vi "Client Test.vi"() -> ()   [LabVIEW 2018]
uses:
  IOPub Messages/status Message/Status Content.ctl
  Shell Messages/kernel_info_request Message/kernel_info_request Message.lvclass
  IOPub Messages/status Message/status Message.lvclass
  Shell Messages/kernel_info_reply Message/kernel_info_reply Message.lvclass
  IOPub Messages/error Message/error Message.lvclass
  Shell Messages/execute_reply Message/execute_reply Message.lvclass
  C:/Users/gavin/Documents/LabVIEW Data/LabVIEW-Bits/Connectivity/Jupyter Client/Base Classes/Reply Message/Reply Message.lvclass
  IOPub Messages/stream Message/stream Message.lvclass
  IOPub Messages/execute_result Message/execute_result Message.lvclass
  C:/Users/gavin/Documents/LabVIEW Data/LabVIEW-Bits/Connectivity/Jupyter Client/IOPub Messages/display_data Message/display_data Message.lvclass
  Shell Messages/shutdown_request Message/shutdown_request Message.lvclass
  Shell Messages/execute_request Message/execute_request Message.lvclass
  48e361d1-6cf2-4824-8834-e089fd543d5e.vi
  48e361d1-6cf2-4824-8834-e089fd543d5e.vi/d7fca688-9f3d-45d2-96bd-b0b513891c02.vi
  48e361d1-6cf2-4824-8834-e089fd543d5e.vi/f5f7bd2d-65e3-4118-a998-9a6677903c6e.vi
  JuPyter_Client/public/Start Kernel and Connect.vi
  <userlib>/_OpenG.lib/lvdata/lvdata.llb/Set Data Name__ogtk.vi
  <userlib>/_OpenG.lib/lvdata/lvdata.llb/Array of VData to VCluster__ogtk.vi
  JuPyter_Client/JuPyter_Client.lvclass
  Base Classes/Message Class/Message Class.lvclass
panel:
  in  "Outputs":T1(tab)
  in  "Streams":enum32{"stdout", "stdeerr"}(tab)
  in  "Cl;ear stdout":bool
  out "Stdout":string
  in  "Cl;ear stderr":bool
  out "stderr":string
  in  "Clear Results":bool
  out "Results":string[](array[string])
  in  "Clear Message":bool
  out "Message Data":string
  in  "Variables to Watch":string[](array[string])
  in  "Enter":bool
  in  "Code":string
  in  "Exit":bool
  out "Language and Version":string
  out "status":T2
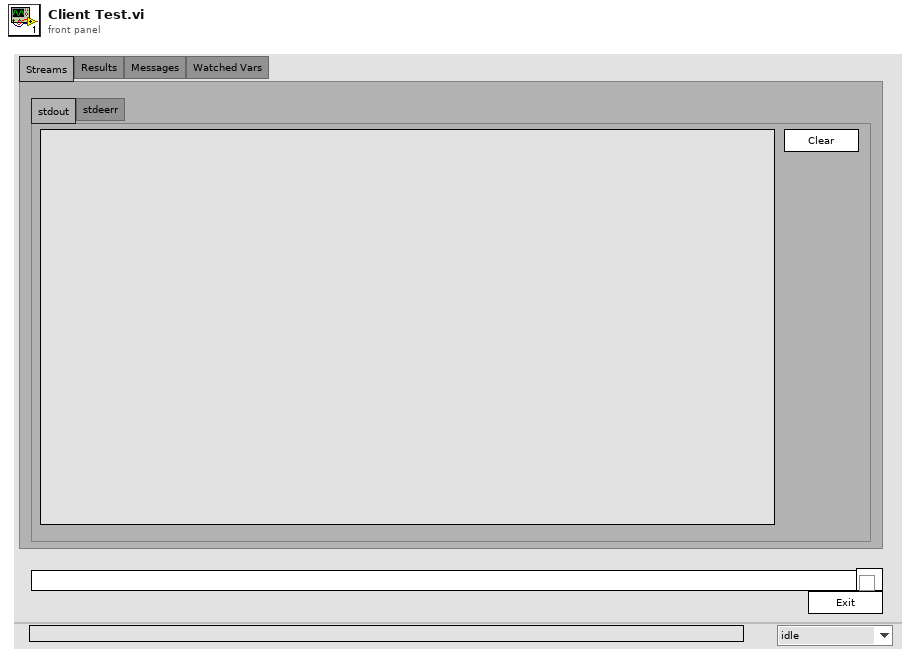
[diagram p1: front panel]
types:
  T1 = enum32{"Streams", "Results", "Messages", "Watched Vars"}
  T2 = typedef "ClientMessaging.lvlib/status Message.lvclass/Status Content.ctl" = enum16{"idle", "busy", "starting"}
  T3 = typedef "ClientMessaging.lvlib/Message Class.lvclass/header_dict.ctl" = cluster{"msg_id":string, "username":string, "session":string, "date":timestamp, "msg_type":string, "version":string}
  T4 = cluster{"ename":string, "evalue":string, "traceback":string[]}
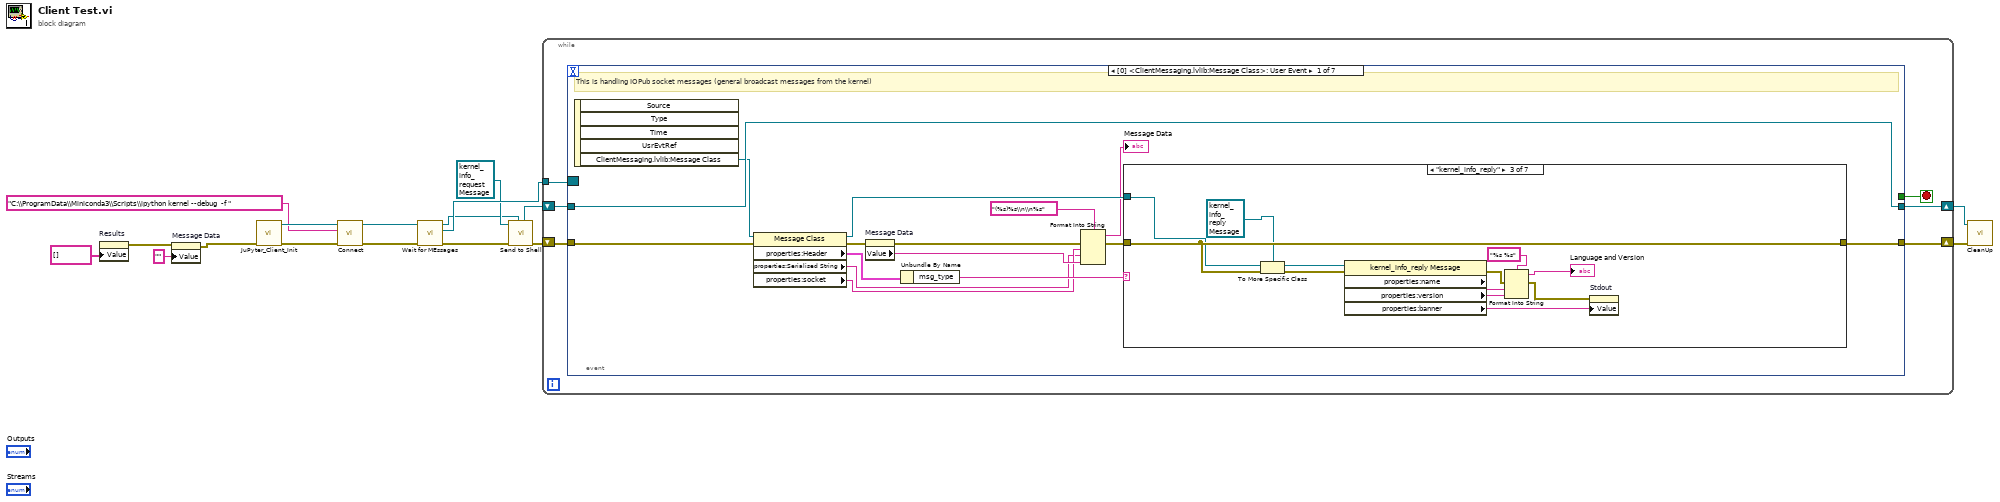
[diagram p0: block diagram]
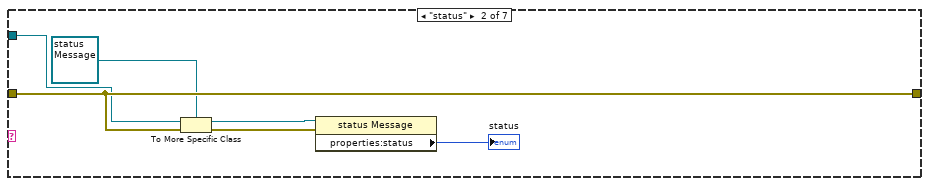
[diagram p3: hidden frame]
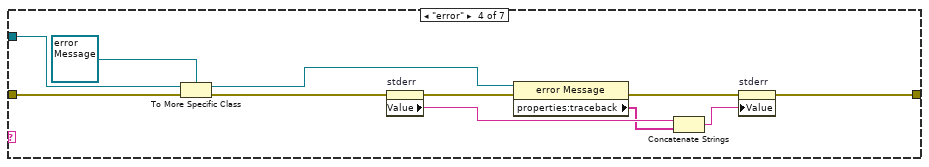
[diagram p4: hidden frame]
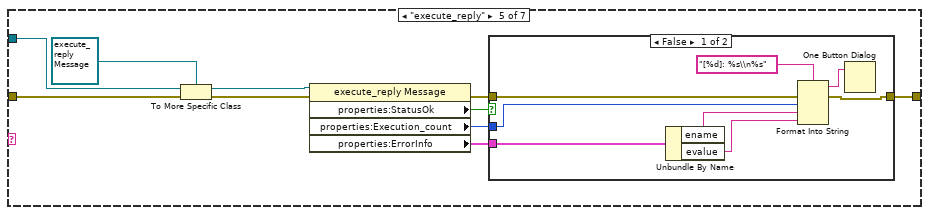
[diagram p5: hidden frame]
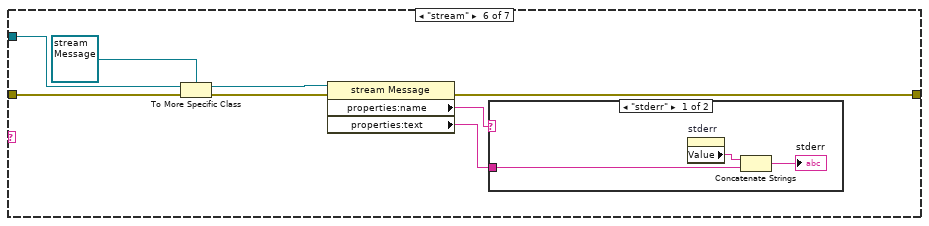
[diagram p7: hidden frame]
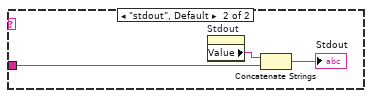
[diagram p8: hidden frame]
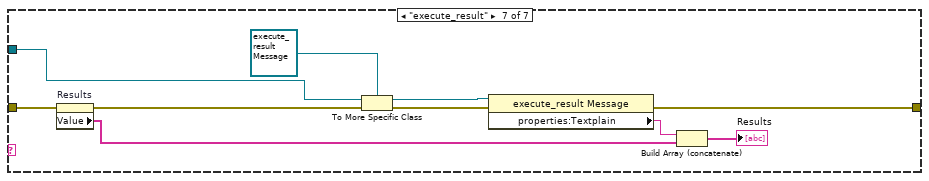
[diagram p9: hidden frame]
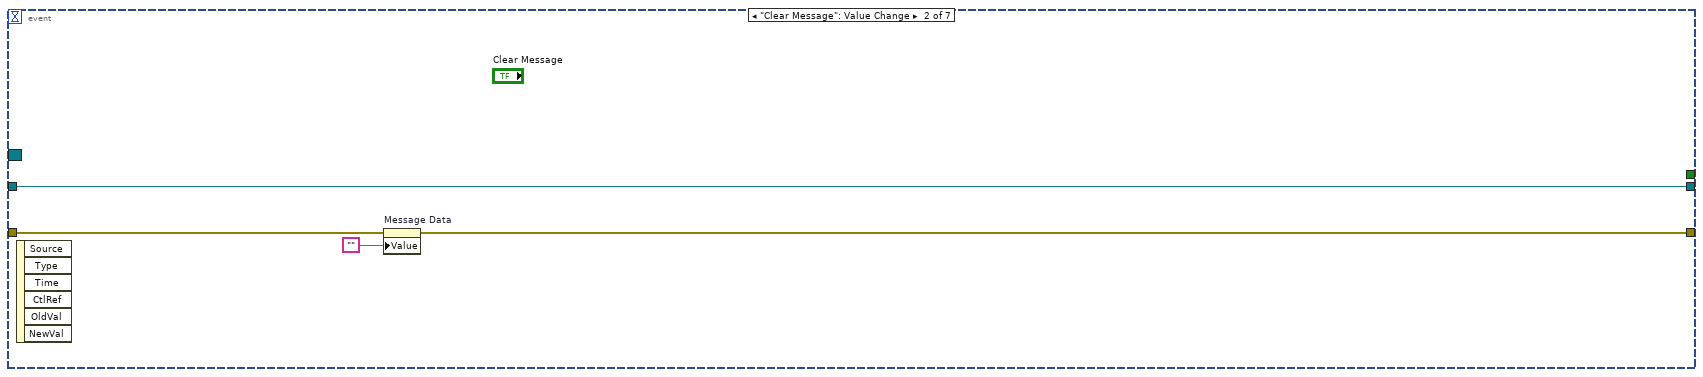
[diagram p10: hidden frame]
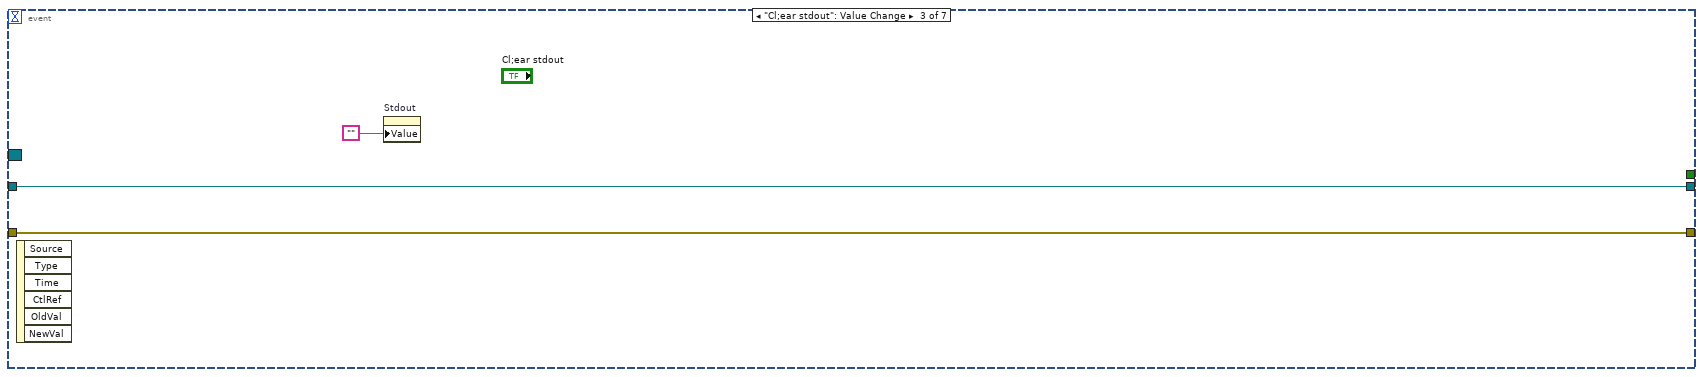
[diagram p11: hidden frame]
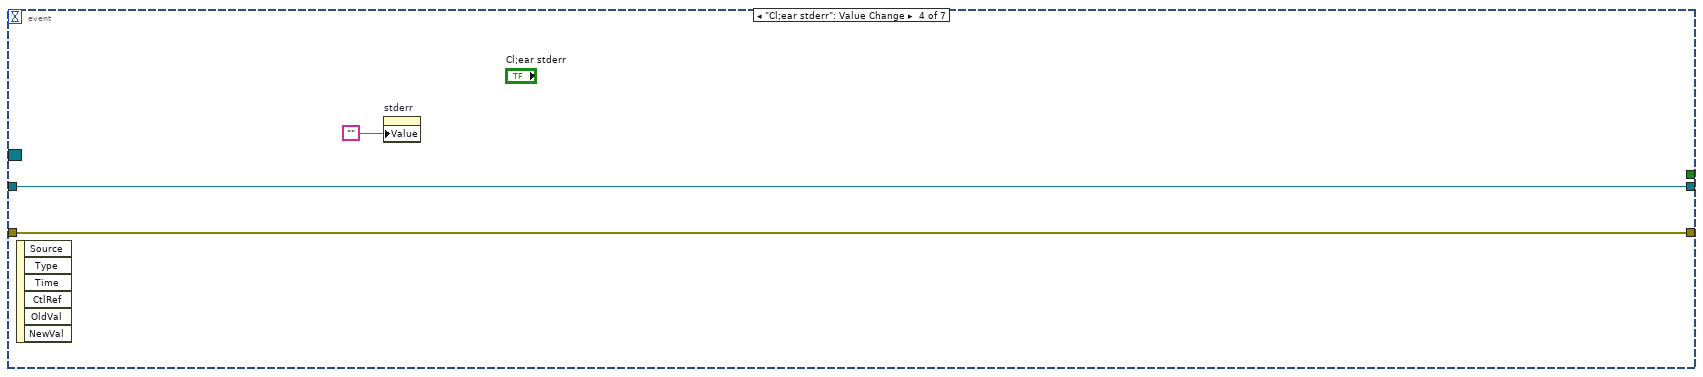
[diagram p12: hidden frame]
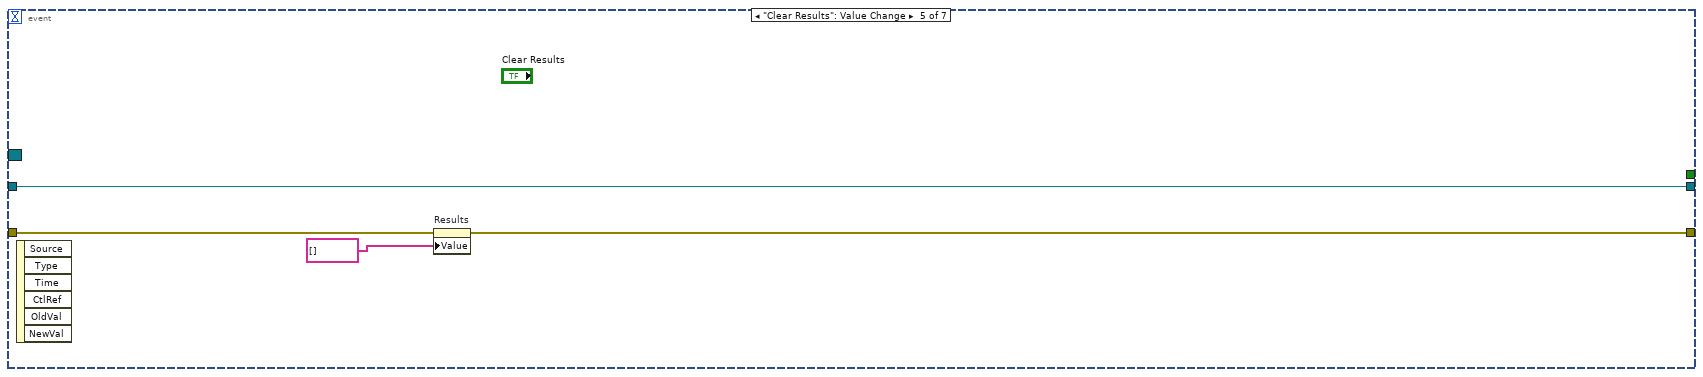
[diagram p13: hidden frame]
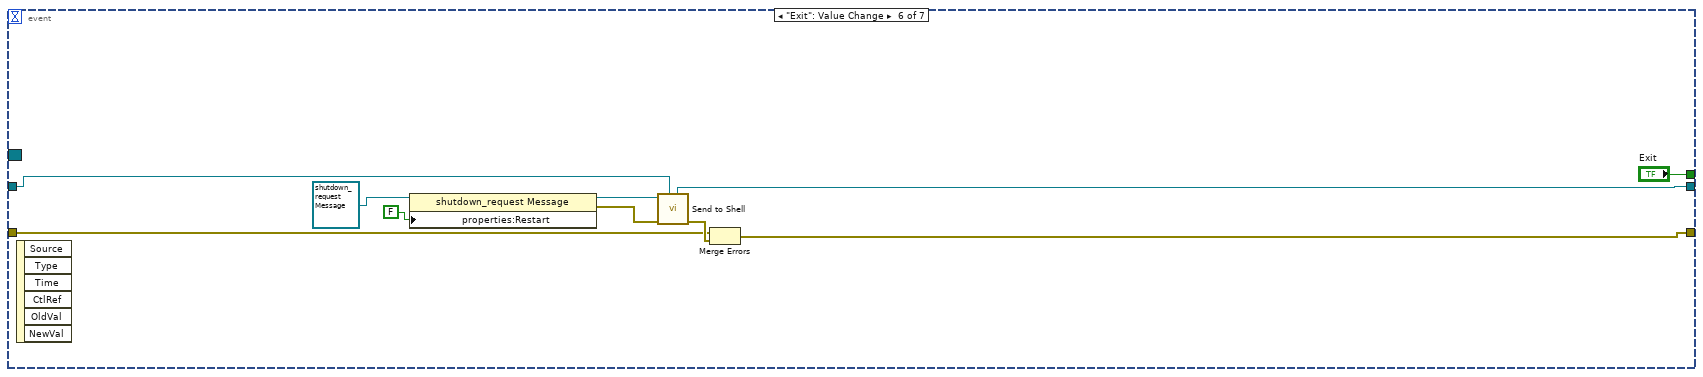
[diagram p14: hidden frame]
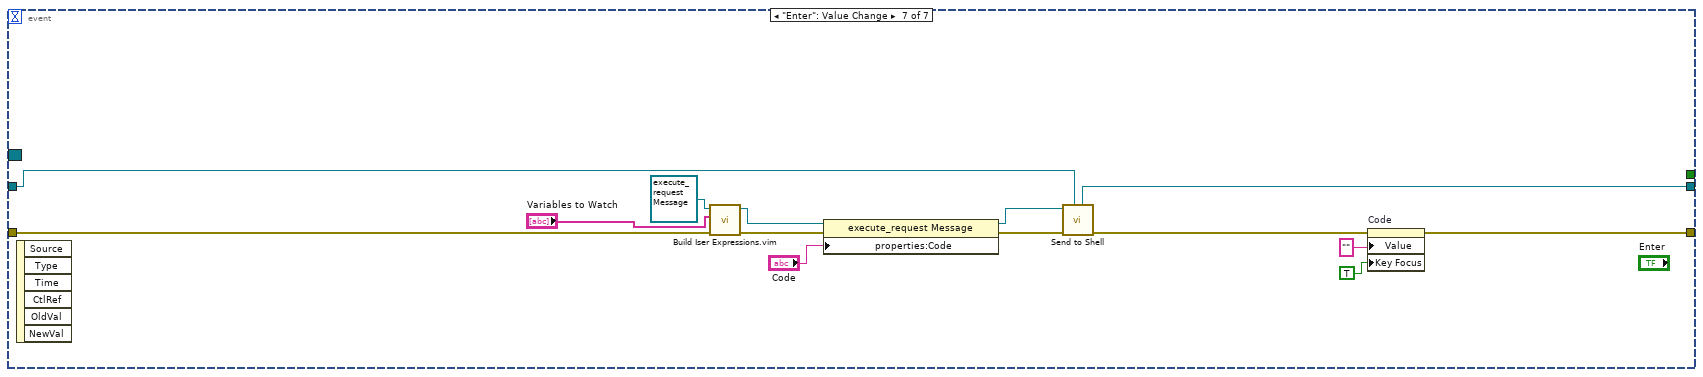
[diagram p15: hidden frame]
diagram:
  n1 = property on="Results" class="Arr (strict)"("Value"=string[] [] ("Results")) -> (error out=w2:errorcluster)  [unwired: 2 in, 1 out]
  n2 = property on="Message Data" class="Str"(error in=w2, "Value"="" ("Message Data")) -> (error out=w3:errorcluster)  [unwired: 1 in, 1 out]
  n3 = call "JuPyter_Client_Init.vi"("error in (no error)"=w3) -> ("error out"=w16:errorcluster, "object out"=w17:refnum<class "JuPyter_Client.lvclass">)  [unwired: 9 in]
  n4 = call-poly "Connect.vi"("error in (no error)"=w16, "Path to Kernel Command (IPython)"="C:\\ProgramData\\Miniconda3\\Scripts\\ipython kernel --debug  -f " ("Command"), "object in"=w17) -> ("error out"=w11:errorcluster, "object out"=w13:refnum<class "JuPyter_Client.lvclass">)  [unwired: 7 in]
  n5 = call-dynamic "Wait for MEssages.vi"("error in (no error)"=w11, "object in"=w13) -> ("error out"=w6:errorcluster, "Event Registration Refnum"=w10:refnum<event-registration>, "object out"=w8:refnum<class "JuPyter_Client.lvclass">)  [unwired: 7 in]
  n6 = call-dynamic "Send to Shell.vi"("Session In"=w8, "error in (no error)"=w6, "object in"=refnum<class "kernel_info_request Message.lvclass"> refnum ("ClientMessaging.lvlib:kernel_info_request Message")) -> ("error out"=w5:errorcluster, "Session Out"=w7:refnum<class "JuPyter_Client.lvclass">)  [unwired: 5 in, 2 out]
  n7 = while {
    shift-right: [w22] -> w15
    shift-left: w7 -> [w19]
    shift-right: [w20] -> w14
    shift-left: w5 -> [w23]
    tunnel: w10 -> [w18]
    stop <- w21 stop-if-true
    n8 = event shown="[0] <ClientMessaging.lvlib:Message Class>: User Event" {
      selector: w18 -> [_ _ _ _ _ _ _]
      dyn-events: _ -> [_ _ _ _ _ _ _]
      timeout: _ -> [_ _ _ _ _ _ _]
      tunnel: w23 -> [w30 w113 w117 w120 w123 w126 w139]
      tunnel: [w36 w115 w118 w121 w125 w132 w145] -> w22
      tunnel: [_ _ _ _ _ "Exit" _] -> w21
      tunnel: [w37 w112 w117 w120 w122 w127 w142] -> w20
      tunnel: w19 -> [w36 w115 w118 w121 w125 w133 w144]
      event User Event {
        # "This is handling IOPub socket messages (general broadcast messages from the kernel)"
        n9 = event-data() -> ("ClientMessaging.lvlib:Message Class"=w31:refnum<class "Message Class.lvclass">)  [unwired: 1 in, 4 out]
        n10 = property class="Message Class"(reference=w31, error in=w30) -> (reference out=w35:refnum<class "Message Class.lvclass">, error out=w28:errorcluster, "properties:Header"=w34:T3, "properties:Serialised String"=w24:string, "properties:socket"=w25:string)
        n11 = property on="Message Data" class="Str"(error in=w28) -> (error out=w27:errorcluster, "Value"=w26:string)  [unwired: 1 in, 1 out]
        n12 = Unbundle By Name(w34) -> ("msg_type"=w38:string)
        n13 = Format Into String(format string="(%s)%s\\n\\n%s", error in=w27, w25, w24, w26) -> (resulting string=→"Message Data":string, error out=w29:errorcluster)  [unwired: 1 in]
        n14 = case shown="\"kernel_info_reply\"" w38 {
          tunnel: w35 -> [_ w43 w56 w67 w77 w95 w110]
          tunnel: w29 -> [w39 w45 w57 w68 w78 w93 w103]
          tunnel: [w39 w45 w57 w58 w69 w90 w111] -> w37
          frame "False", Default {
          }
          frame "status" {
            n15 = To More Specific Class(target class=refnum<class "status Message.lvclass"> refnum ("ClientMessaging.lvlib:status Message"), reference=w43, error in=w45) -> (specific class reference=w42:refnum<class "status Message.lvclass">, error out=w41:errorcluster)
            n16 = property class="status Message"(reference=w42, error in=w41) -> ("properties:status"=→"status":T2)  [unwired: 2 out]
          }
          frame "kernel_info_reply" {
            n17 = To More Specific Class(target class=refnum<class "kernel_info_reply Message.lvclass"> refnum ("ClientMessaging.lvlib:kernel_info_reply"), reference=w56, error in=w57) -> (specific class reference=w55:refnum<class "kernel_info_reply Message.lvclass">, error out=w54:errorcluster)
            n18 = property class="kernel_info_reply Message"(reference=w55, error in=w54) -> (error out=w51:errorcluster, "properties:name"=w50:string, "properties:version"=w49:string, "properties:banner"=w46:string)  [unwired: 1 out]
            n19 = Format Into String(format string="%s %s", error in=w51, w50, w49) -> (resulting string=→"Language and Version":string, error out=w47:errorcluster)  [unwired: 1 in]
            n20 = property on="Stdout" class="Str"(error in=w47, "Value"=w46) -> ()  [unwired: 1 in, 2 out]
          }
          frame "error" {
            n21 = To More Specific Class(target class=refnum<class "error Message.lvclass"> refnum ("ClientMessaging.lvlib:error Message"), reference=w67, error in=w68) -> (specific class reference=w66:refnum<class "error Message.lvclass">, error out=w61:errorcluster)
            n22 = property on="stderr" class="Str"(error in=w61) -> (error out=w60:errorcluster, "Value"=w64:string)  [unwired: 1 in, 1 out]
            n23 = property class="error Message"(reference=w66, error in=w60) -> (error out=w59:errorcluster, "properties:traceback"=w63:string[])  [unwired: 1 out]
            n24 = Concatenate Strings(w64, w63) -> (w62:string)
            n25 = property on="stderr" class="Str"(error in=w59, "Value"=w62) -> (error out=w58:errorcluster)  [unwired: 1 in, 1 out]
          }
          frame "execute_reply" {
            n26 = To More Specific Class(target class=refnum<class "execute_reply Message.lvclass"> refnum ("ClientMessaging.lvlib:execute_reply Message"), reference=w77, error in=w78) -> (specific class reference=w76:refnum<class "execute_reply Message.lvclass">, error out=w71:errorcluster)
            n27 = property class="execute_reply Message"(reference=w76, error in=w71) -> (error out=w70:errorcluster, "properties:StatusOk"=w74:bool, "properties:Execution_count"=w73:u32, "properties:ErrorInfo"=w72:T4)  [unwired: 1 out]
            n28 = case shown="False" w74 {
              tunnel: w73 -> [w84 _]
              tunnel: w72 -> [w86 _]
              tunnel: w70 -> [w80 w87]
              tunnel: [w79 w87] -> w69
              frame False {
                n29 = Unbundle By Name(w86) -> ("ename"=w83:string, "evalue"=w82:string)
                n30 = Format Into String(format string="[%d]: %s\\n%s", error in=w80, w84, w83, w82) -> (resulting string=w81:string, error out=w79:errorcluster)  [unwired: 1 in]
                n31 = One Button Dialog(message=w81) -> ()  [unwired: 1 in, 1 out]
              }
              frame True {
              }
            }
          }
          frame "stream" {
            n32 = To More Specific Class(target class=refnum<class "stream Message.lvclass"> refnum ("ClientMessaging.lvlib:stream Message"), reference=w95, error in=w93) -> (specific class reference=w92:refnum<class "stream Message.lvclass">, error out=w91:errorcluster)
            n33 = property class="stream Message"(reference=w92, error in=w91) -> (error out=w90:errorcluster, "properties:name"=w89:string, "properties:text"=w88:string)  [unwired: 1 out]
            n34 = case shown="\"stderr\"" w89 {
              tunnel: w88 -> [w97 w100]
              frame "stderr" {
                n35 = property on="stderr" class="Str"() -> ("Value"=w98:string)  [unwired: 2 in, 2 out]
                n36 = Concatenate Strings(w98, w97) -> (→"stderr":string)
              }
              frame "stdout", Default {
                n37 = property on="Stdout" class="Str"() -> ("Value"=w101:string)  [unwired: 2 in, 2 out]
                n38 = Concatenate Strings(w101, w100) -> (→"Stdout":string)
              }
            }
          }
          frame "execute_result" {
            n39 = property on="Results" class="Arr (strict)"(error in=w103) -> (error out=w102:errorcluster, "Value"=w104:string[])  [unwired: 1 in, 1 out]
            n40 = To More Specific Class(target class=refnum<class "execute_result Message.lvclass"> refnum ("ClientMessaging.lvlib:execute_result Message"), reference=w110, error in=w102) -> (specific class reference=w108:refnum<class "execute_result Message.lvclass">, error out=w107:errorcluster)
            n41 = property class="execute_result Message"(reference=w108, error in=w107) -> (error out=w111:errorcluster, "properties:Textplain"=w106:string)  [unwired: 1 out]
            n42 = Build Array (concatenate)(w106, w104) -> (→"Results":string[])
          }
        }
      }
      event "Clear Message": Value Change {
        n43 = event-data() -> ()  [unwired: 1 in, 6 out]
        n44 = property on="Message Data" class="Str"(error in=w113, "Value"="") -> (error out=w112:errorcluster)  [unwired: 1 in, 1 out]
      }
      event "Cl;ear stdout": Value Change {
        n45 = event-data() -> ()  [unwired: 1 in, 6 out]
        n46 = property on="Stdout" class="Str"("Value"="") -> ()  [unwired: 2 in, 2 out]
      }
      event "Cl;ear stderr": Value Change {
        n47 = event-data() -> ()  [unwired: 1 in, 6 out]
        n48 = property on="stderr" class="Str"("Value"="") -> ()  [unwired: 2 in, 2 out]
      }
      event "Clear Results": Value Change {
        n49 = event-data() -> ()  [unwired: 1 in, 6 out]
        n50 = property on="Results" class="Arr (strict)"(error in=w123, "Value"=string[] [] ("Results")) -> (error out=w122:errorcluster)  [unwired: 1 in, 1 out]
      }
      event "Exit": Value Change {
        n51 = event-data() -> ()  [unwired: 1 in, 6 out]
        n52 = property class="shutdown_request Message"(reference=refnum<class "shutdown_request Message.lvclass"> refnum ("ClientMessaging.lvlib:shutdown_request Message"), "properties:Restart"=FALSE ("Restart")) -> (reference out=w130:refnum<class "shutdown_request Message.lvclass">, error out=w129:errorcluster)  [unwired: 1 in]
        n53 = call-dynamic "Send to Shell.vi"("Session In"=w133, "error in (no error)"=w129, "object in"=w130) -> ("error out"=w131:errorcluster, "Session Out"=w132:refnum<class "JuPyter_Client.lvclass">)  [unwired: 5 in, 2 out]
        n54 = Merge Errors(w126, w131) -> (w127:errorcluster)
      }
      event "Enter": Value Change {
        n55 = event-data() -> ()  [unwired: 1 in, 6 out]
        n56 = call "Build Iser Expressions.vim"("error in (no error)"=w139, "List of variables to return"="Variables to Watch", "object in"=refnum<class "execute_request Message.lvclass"> refnum ("ClientMessaging.lvlib:execute_request Message")) -> ("error out"=w140:errorcluster, "object out"=w141:refnum<class "execute_request Message.lvclass">)  [unwired: 7 in]
        n57 = property class="execute_request Message"(reference=w141, error in=w140, "properties:Code"="Code") -> (reference out=w147:refnum<class "execute_request Message.lvclass">, error out=w146:errorcluster)
        n58 = call-dynamic "Send to Shell.vi"("Session In"=w144, "error in (no error)"=w146, "object in"=w147) -> ("error out"=w136:errorcluster, "Session Out"=w145:refnum<class "JuPyter_Client.lvclass">)  [unwired: 5 in, 2 out]
        n59 = property on="Code" class="Str"(error in=w136, "Value"="" ("Code"), "Key Focus"=TRUE) -> (error out=w142:errorcluster)  [unwired: 1 in, 1 out]
      }
    }
  }
  n60 = call-dynamic "CleanUp.vi"("error in (no error)"=w14, "object in"=w15) -> ()  [unwired: 8 in, 2 out]
